vi "Add Word.vi"(8 "error in":errorcluster, 10 "name (Word)":string="Word", 11 "label ref":T1 format="%.0x") -> (0 "error out":errorcluster, 1 "newly created?":bool, 2 "word ref":T1 format="%.0x", 3 "label ref out":T1 format="%.0x")   [LabVIEW 2020, in "AIM ARINC 429 Scripting.lvlib"]
uses:
  AIM ARINC 429 Scripting.lvlib
  <vilib>/NI VeriStand/Custom Device API/Custom Device Item Ref.ctl
  Constants.vi
  <vilib>/NI VeriStand/Custom Device API/Custom Device API.lvlib
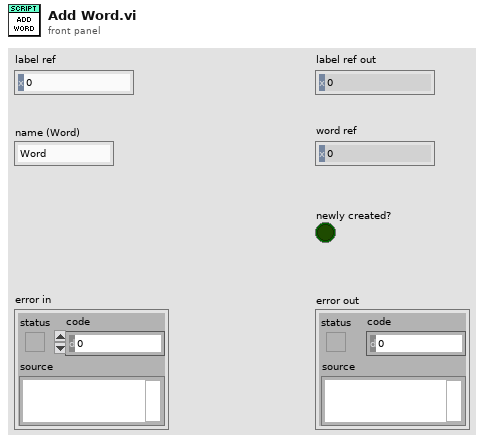
[diagram p1: front panel]
types:
  T1 = typedef "Custom Device API.lvlib/Custom Device Item Ref.ctl" = u64
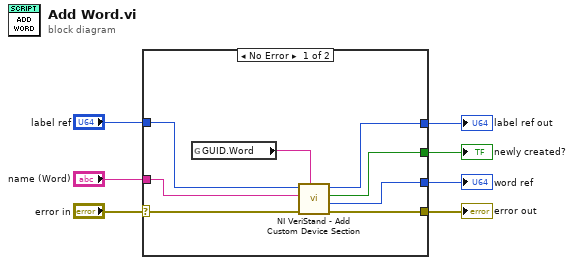
[diagram p0: block diagram]
diagram:
  n1 = case shown="No Error" "error in" {
    selector: "error in" -> [w15 w17]
    tunnel: [w14 w17] -> w6
    tunnel: "label ref" -> [w12 w16]
    tunnel: [w11 _] -> w4
    tunnel: "name (Word)" -> [w13 _]
    tunnel: [w10 _] -> w2
    tunnel: [w9 w16] -> w1
    frame No Error {
      n2 = global read "Constants.vi" "GUID.Word"() -> (w8:string)
      n3 = call <vilib>:"NI VeriStand - Add Custom Device Section.vi"("GUID (Default Section)"=w8, "error in (no error)"=w15, "Section Name"=w13, "Parent Ref in"=w12) -> ("error out"=w14:errorcluster, "Section Ptr"=w11:T1, "Newly Created?"=w10:bool, "Parent Ref out"=w9:T1)  [unwired: 4 in]
    }
    frame Error {
    }
  }
  "word ref" <- w4
  "error out" <- w6
  "newly created?" <- w2
  "label ref out" <- w1
